vi "snap_with_gain.vi"(6 "Optional ROI":u32[](array[numeric])=[0, 0, 32767, 32767], 7 "Optional Binning":u32, 8 "error in (no error)":errorcluster, 9 "Optional Gain":u32, 10 "Optional Exposure":u32, 11 "New Image":T1) -> (0 "error out":errorcluster, 1 "Gain out":u32, 2 "Exposure out":u32, 3 "Image Out":T1, 4 "ROI out":u32[](array[numeric])=[0, 0, 32767, 32767], 5 "Binning out":u32)   [LabVIEW 2011]
doc: "Snap an image. This VI opens the first available camera, captures an image, and closes the camera.\n\nImage: an IMAQ image\nOptional exposure: in microseconds.\nOptional binning: pixel binning, usually from 1 to 4\nOptional ROI: array of {x, y, width, height}\n\nThe actual exposure, binning, and ROI values are output."
uses:
  <vilib>/vision/Image Controls.llb/IMAQ Image.ctl
panel:
  out "dT":u32
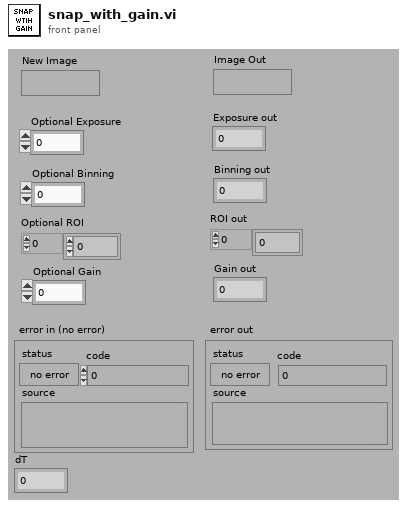
[diagram p1: front panel]
types:
  T1 = typedef "IMAQ Image.ctl" = refnum<image>
  T2 = enum32{"gain", "offset", "exposure", "binning", "horizontal binning", "vertical binning", "readout speed", "trigger type", "lcd filter", "cooler", "exposure red", "exposure blue", "image format", "roi x", "roi y", "roi width", "roi height", "reserved1", "shutter state", "reserved2", "sync-b out", "reserved3", "intensifier gain", "trigger delay", "camera mode", "normalized gain", "normalized intenifier gain DB", "doPostProcessing", "postProcessGainRed", "postProcessGainGreen", "postProcessGainBlue", "postProcessBayerAlgorithm", "postProcessImageFormat", "fan", "blackout mode", "high sensitivity", "Readout Port", "EM Gain", "open delay", "close delay", "clearing mode"}
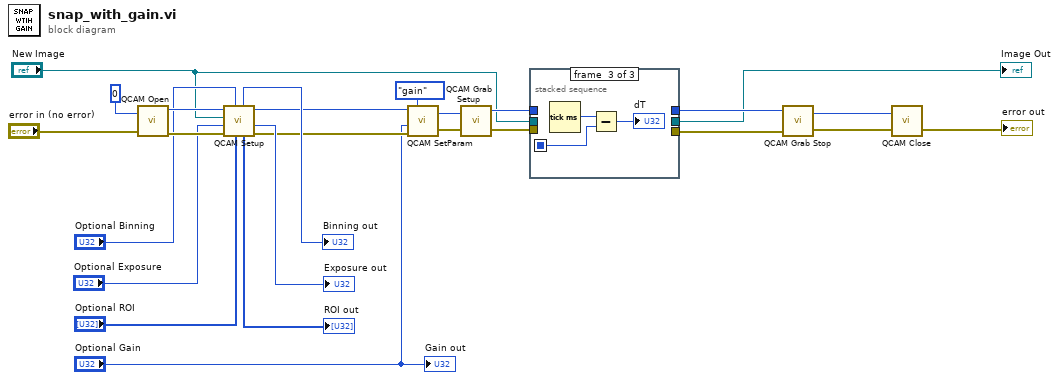
[diagram p0: block diagram]
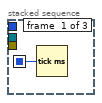
[diagram p2: hidden frame]
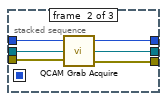
[diagram p3: hidden frame]
diagram:
  n1 = call <userlib>:"QCAM Open.vi"("error in (no error)"="error in (no error)", "cameraId"=0) -> ("error out"=w18:errorcluster, "cameraId out"=w25:u32)
  n2 = call <userlib>:"QCAM Setup.vi"("Optional ROI"="Optional ROI", "Optional Binning"="Optional Binning", "error in (no error)"=w18, "Optional Exposure"="Optional Exposure", "Image"="New Image", "cameraId"=w25) -> ("error out"=w6:errorcluster, "Exposure out"=→"Exposure out":u32, "cameraId out"=w2:u32, "ROI out"=→"ROI out":u32[], "Binning out"=→"Binning out":u32)  [unwired: 1 in]
  n3 = call <userlib>:"QCAM SetParam.vi"("error in (no error)"=w6, "value"="Optional Gain", "parameter key"=T2."gain", "cameraId"=w2) -> ("error out"=w5:errorcluster, "cameraId out"=w4:u32)
  n4 = call <userlib>:"QCAM Grab Setup.vi"("error in (no error)"=w5, "cameraId"=w4) -> ("error out"=w19:errorcluster, "cameraId out"=w24:u32)
  n5 = stacked-sequence {
    seq-local: [w26 _ _] -> [_ _ w34]
    tunnel: w24 -> [_ w32 _]
    tunnel: [_ w31 _] -> w23
    tunnel: [_ w30 _] -> w20
    tunnel: w19 -> [_ w29 _]
    tunnel: [_ w28 _] -> w9
    tunnel: "New Image" -> [_ w27 _]
    frame #0 {
      n6 = Tick Count (ms)() -> (millisecond timer value=w26:u32)
    }
    frame #1 {
      n7 = call <userlib>:"QCAM Grab Acquire.vi"("error in (no error)"=w29, "Image"=w27, "cameraId"=w32) -> ("error out"=w30:errorcluster, "Image Out"=w28:T1, "cameraId out"=w31:u32)
    }
    frame #2 {
      n8 = Tick Count (ms)() -> (millisecond timer value=w35:u32)
      n9 = Subtract(x=w35, y=w34) -> (x-y=→"dT":u32)
    }
  }
  "Image Out" <- w9
  n10 = call <userlib>:"QCAM Grab Stop.vi"("error in (no error)"=w20, "cameraId"=w23) -> ("error out"=w21:errorcluster, "cameraId Out"=w22:u32)
  n11 = call <userlib>:"QCAM Close.vi"("error in (no error)"=w21, "cameraId"=w22) -> ("error out"=→"error out":errorcluster)  [unwired: 1 in]
  "Gain out" <- "Optional Gain"
